vi "Save map as png.vi"(4 "error in":errorcluster, 5 "input main cluster":T1) -> (0 "error out":errorcluster, 1 "output main cluster":T1)   [LabVIEW 2010]
uses:
  Main_cluster.ctl
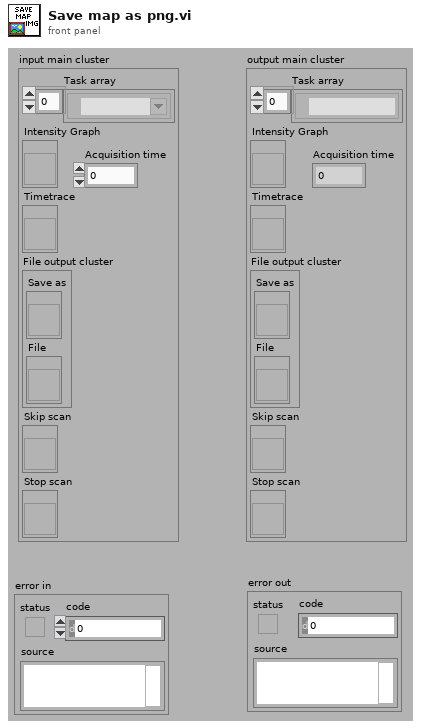
[diagram p1: front panel]
types:
  T1 = typedef "Main_cluster.ctl" = cluster{"Task array":refnum<k21>[], "Intensity Graph":refnum<vi>, "Timetrace":refnum<vi>, "File output cluster":cluster{"Save as":refnum<vi>, "File":refnum<vi>}, "Skip scan":refnum<vi>, "Stop scan":refnum<vi>, "Acquisition time":dbl}
  T2 = typedef "imagedata.ctl" = cluster{"image type":i32, "image depth":i32, "image":u8[], "mask":u8[], "colors":u32[], "Rectangle":cluster{"left":i16, "top":i16, "right":i16, "bottom":i16}}
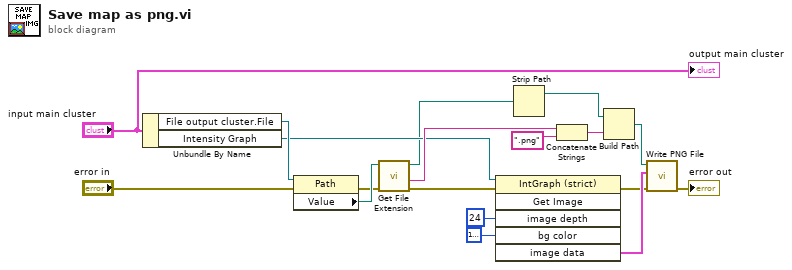
[diagram p0: block diagram]
diagram:
  n1 = Unbundle By Name("input main cluster") -> ("File output cluster.File"=w7:refnum<vi>, "Intensity Graph"=w3:refnum<vi>)
  n2 = property class="Path"(reference=w7, error in="error in") -> (error out=w4:errorcluster, "Value"=w6:path)  [unwired: 1 out]
  n3 = call <vilib>:"Get File Extension.vi"("error in (no error)"=w4, "file"=w6) -> ("error out"=w16:errorcluster, "filename without extension"=w10:string, "dup file"=w1:path)  [unwired: 6 in, 1 out]
  n4 = invoke on="Invoke Node" class="IntGraph (strict)" method="Get Image"(reference=w3, error in=w16, "image depth"=24 ("Image Depth"), "bg color"=u32 16777226 ("Background Color")) -> (error out=w12:errorcluster, "image data"=w15:T2)  [unwired: 2 in, 4 out]
  n5 = Strip Path(path=w1) -> (stripped path=w11:path)  [unwired: 1 out]
  n6 = Concatenate Strings(w10, ".png" ("string")) -> (w8:string)
  n7 = Build Path(base path=w11, name or relative path=w8) -> (appended path=w17:path)
  n8 = call <vilib>:"Write PNG File.vi"("error in (no error)"=w12, "image data"=w15, "path to PNG file"=w17) -> ("error out"=→"error out":errorcluster)  [unwired: 7 in, 1 out]
  "output main cluster" <- "input main cluster"
